vi "GetkA(34401A) v0.5.vi"(0 "GPIB Address":u32=6 max=31 step=1, 1 "error in":errorcluster) -> (2 "Voltage (V)":dbl=6.0373e-05 format="%.7f", 3 "Curent (kA)":dbl=0.000241492 format="%.7f", 4 "error out":errorcluster)   [LabVIEW 2020]
panel:
  in  "HP 34401A GPIB":string="8"
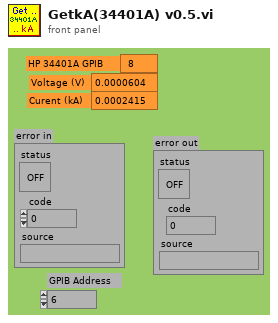
[diagram p1: front panel]
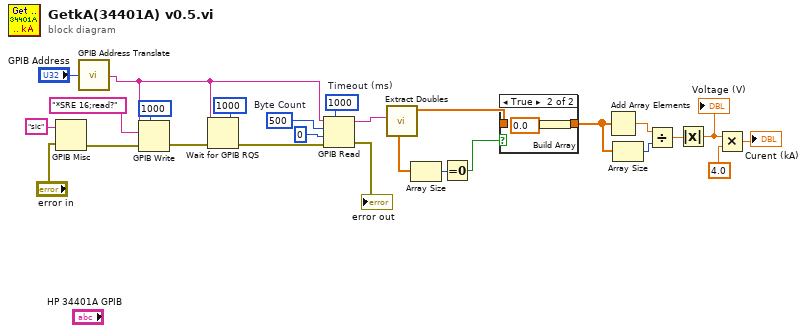
[diagram p0: block diagram]
diagram:
  w10 = 500  # Byte Count
  w11 = 1000  # Timeout (ms)
  n1 = GPIB Misc(0:"sic", 1:"error in") -> (4:w9:errorcluster)  [unwired: 2 out]
  n2 = call "GPIB Address Translate.vi"("GPIB Address"="GPIB Address") -> ("GPIB Address String"=w2:string)
  n3 = GPIB Write(0:w2, 1:"*SRE 16;read?", 3:w9, 4:u32 1000) -> (6:w8:errorcluster)  [unwired: 1 in, 1 out]
  n4 = Wait for GPIB RQS(2:w8, 3:u32 1000, 4:w2) -> (0:w7:errorcluster)  [unwired: 1 out]
  n5 = GPIB Read(0:w2, 1:w10, 2:0 ("Mode"), 3:w7, 4:w11) -> (5:w13:string, 7:→"error out":errorcluster)  [unwired: 1 out]
  n6 = call "Extract Doubles.vi"("String"=w13) -> ("Data"=w16:dbl[])  [unwired: 5 in, 1 out]
  n7 = Array Size(array=w16) -> (size(s)=w15:i32)
  n8 = Equal To 0?(x=w15) -> (x = 0?=w14:bool)
  n9 = case shown="True" w14 {
    tunnel: [w26 w27] -> w25
    tunnel: w16 -> [w26 _]
    frame False {
    }
    frame True {
      n10 = Build Array(0.0) -> (w27:dbl[])
    }
  }
  n11 = Add Array Elements(numeric array=w25) -> (sum=w24:dbl)
  n12 = Array Size(array=w25) -> (size(s)=w23:i32)
  n13 = Divide(x=w24, y=w23) -> (x/y=w5:dbl)
  n14 = Absolute Value(x=w5) -> (abs(x)=w4:dbl)
  "Voltage (V)" <- w4
  n15 = Multiply(x=w4, y=4.0) -> (x*y=→"Curent (kA)":dbl)
